vi "FringeTrackerTrack.vi"(6 "error in (no error)":errorcluster, 9 "FringeTracker Name":string="TipTiltMirror[1]") -> (0 "error out":errorcluster caption="error in (no error)", 3 "FringeTracker Name out":string)   [LabVIEW 2009]
uses:
  lib/lvrtc.dll
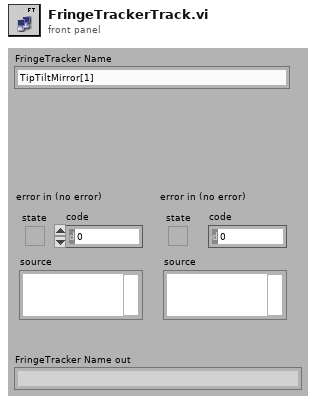
[diagram p1: front panel]
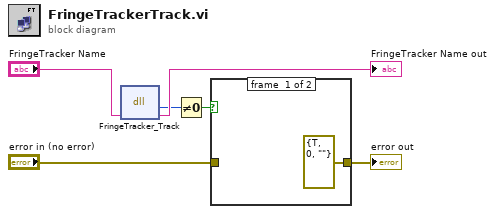
[diagram p0: block diagram]
diagram:
  n1 = dll-call lib="C:/Ohana/LV2009/OhanaOS-LV81/Instruments/RTC/Api/lib/lvrtc.dll" fn="FringeTracker_Track"("FringeTrackerName"="FringeTracker Name") -> ("return type"=w3:i32, "FringeTrackerName"=→"FringeTracker Name out":string)  [unwired: 3 in, 2 out]
  n2 = Not Equal To 0?(x=w3) -> (x != 0?=w2:bool)
  n3 = case shown="False" w2 {
    tunnel: "error in (no error)" -> [_ w8]
    tunnel: [errorcluster {"status"=TRUE, "code"=0, "source"=""} ("error in (no error)") w8] -> w1
    frame #0 {
    }
    frame #1 {
    }
  }
  "error out" <- w1
